vi "Do.vi"(8 "error in":errorcluster, 10 "Actor in":refnum<class "Actor.lvclass">, 11 "Update TE Tech Heating Params":refnum<class "Update TE Tech Heating Params.lvclass">) -> (0 "error out":errorcluster, 2 "Actor out":refnum<class "Actor.lvclass">)   [LabVIEW 2014, in "Controller.lvlib" / "Update TE Tech Heating Params.lvclass"]
doc: "(<B>Filename</B>: Actor Framework.lvlib:Message.lvclass:Do.vi)\n\nDefines what a message does when it is received by an actor. Generally, a message instructs an actor to invoke one of its methods. By default, this method does nothing. A child class must override it to define behavior. Create a child class by using the Actor Framework Message Maker dialog box."
uses:
  Update TE Tech Heating Params.lvclass
  <vilib>/ActorFramework/Actor/Actor.lvclass
  Controller.lvclass
  Controls/eMap.ctl
  <vilib>/ActorFramework/Message Enqueuer/Message Enqueuer.lvclass
  Controller.lvclass/Controller.ctl
  SuperActor/SuperActor.lvclass/SuperActor.ctl
  Update TE Tech Heating Params.lvclass/Update TE Tech Heating Params.ctl
  Update TEC Multipliers/Update TEC Multipliers.lvclass
  Update TEC Multipliers/Update TEC Multipliers.lvclass/Update TEC Multipliers.ctl
  <vilib>/ActorFramework/Message Enqueuer/Message Enqueuer.lvclass/Message Enqueuer.ctl
  Update TEC Multipliers/Write htx.vi
  Accessors/Read Enqueuer Map.vi
  SuperActor/Read Log Session.vi
  <vilib>/ActorFramework/Message Priority Queue/Priority Enqueue.vi
  <userlib>/_Session Fwk/Session - Root.lvclass
  reusable/Session APIs/Session Log/System Log.lvclass
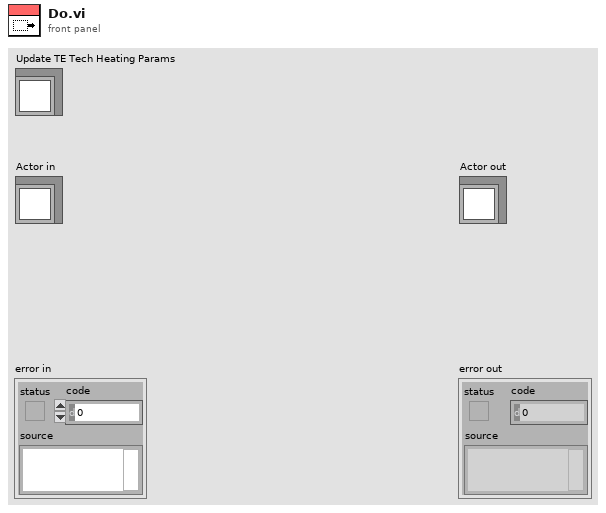
[diagram p1: front panel]
types:
  T1 = typedef "Controller.lvlib/Controller.lvclass/eMap.ctl" = cluster{"Enqueuer":refnum<class "Message Enqueuer.lvclass">, "Active":bool}
  T2 = typedef "Session - Root.lvclass/Session Handle.ctl" = refnum<data-value>
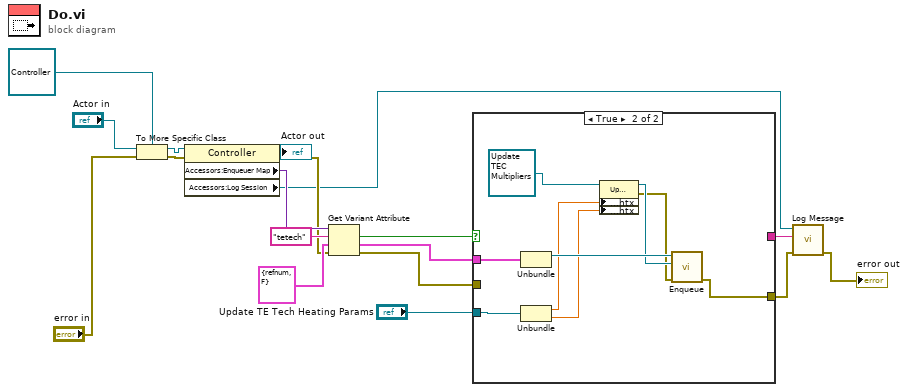
[diagram p0: block diagram]
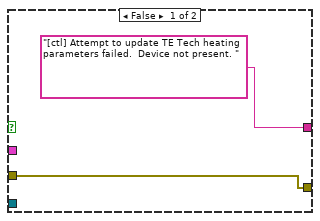
[diagram p2: hidden frame]
diagram:
  n1 = To More Specific Class(target class=refnum<class "Controller.lvclass"> refnum ("Controller:Controller"), reference="Actor in", error in="error in") -> (specific class reference=w16:refnum<class "Controller.lvclass">, error out=w10:errorcluster)
  n2 = property class="Controller"(reference=w16, error in=w10) -> (reference out=→"Actor out":refnum<class "Controller.lvclass">, error out=w9:errorcluster, "Accessors:Enqueuer Map"=w14:variant, "Accessors:Log Session"=w4:T2)
  n3 = Get Variant Attribute(Variant=w14, name="tetech", default value (empty Variant)=T1 {"Enqueuer"=refnum, "Active"=FALSE} ("eMap"), error in=w9) -> (found=w8:bool, value=w7:T1, error out=w6:errorcluster)  [unwired: 1 out]
  n4 = case shown="True" w8 {
    tunnel: w7 -> [_ w29]
    tunnel: w6 -> [w20 _]
    tunnel: "Update TE Tech Heating Params" -> [_ w27]
    tunnel: [w20 w22] -> w3
    tunnel: ["[ctl] Attempt to update TE Tech heating parameters failed.  Device not present. " _] -> w1
    frame False {
    }
    frame True {
      n5 = Unbundle(w29) -> ("Enqueuer"=w28:refnum<class "Message Enqueuer.lvclass">)  [unwired: 1 out]
      n6 = Unbundle(w27) -> (w26:dbl, w25:dbl)
      n7 = property class="Update TEC Heating Params"(reference=refnum<class "Update TEC Multipliers.lvclass"> refnum ("TE Cooler.lvlib:Update TEC PID"), "Accessors:htx"=w26, "Accessors:htx"=w25) -> (reference out=w24:refnum<class "Update TEC Multipliers.lvclass">, error out=w23:errorcluster)  [unwired: 1 in]
      n8 = call <vilib>:"Enqueue.vi"("error in (no error)"=w23, "Message"=w24, "Message Enqueuer in"=w28) -> ("error out"=w22:errorcluster)  [unwired: 7 in, 1 out]
    }
  }
  n9 = call "Log Message.vi"("error in"=w3, "MSG In"=w1, "session in"=w4) -> ("error out"=→"error out":errorcluster)  [unwired: 7 in, 1 out]
